vi "dummy_read.vi"(4 "ViStatusOut 2":T2, 5 "InterfaceInfoOut 2":T1, 6 "SyncType3000":enum16{"none", "TTL", "TTL_kadr", "analog"}(ring), 7 "Ctrl Reference":refnum<vi>) -> (0 "ViStatusOut":T2, 2 "InterfaceInfoOut":T1)   [LabVIEW 2010]
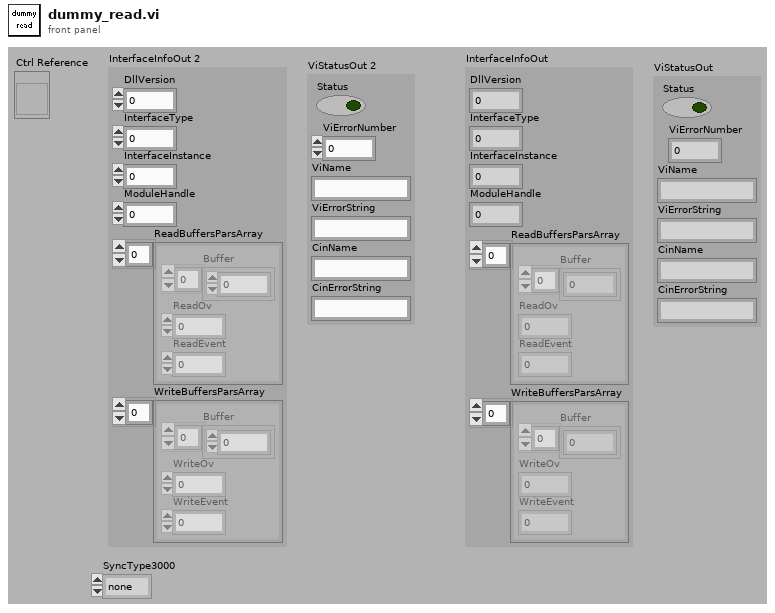
[diagram p1: front panel]
types:
  T1 = cluster{"DllVersion":u32, "InterfaceType":u32, "InterfaceInstance":u32, "ModuleHandle":u32, "ReadBuffersParsArray":cluster{"Buffer":i16[], "ReadOv":u32, "ReadEvent":u32}[], "WriteBuffersParsArray":cluster{"Buffer":i16[], "WriteOv":u32, "WriteEvent":u32}[]}
  T2 = cluster{"Status":bool, "ViErrorNumber":u32, "ViName":string, "ViErrorString":string, "CinName":string, "CinErrorString":string}
  T3 = cluster{"size":u16, "InputEnabled":bool, "CorrectionEnabled":bool, "InputClockSource":u16, "InputType":u16, "SynchroType":u16, "SynchroAdType":u16, "SynchroAdMode":u16, "SynchroAdChannel":u16, "SynchroAdPorog":i16, "ChannelsQuantity":u16, "ControlTable":u16[], "InputFifoBaseAddress":u16, "InputFifoLength":u16, "InputRate":dbl, "InterKadrDelay":dbl, "ChannelRate":dbl, "AdcOffsetCoefArray":dbl[], "AdcScaleCoefArray":dbl[], "BuffersLengthArray":u32[]}
  T4 = cluster{"index":i32, "BufferLength":u32, "RequestStatus":bool}
  T5 = cluster{"ReadBufferIndex":u32, "NumberOfWordsToRead":u32, "RequestStatus":bool}
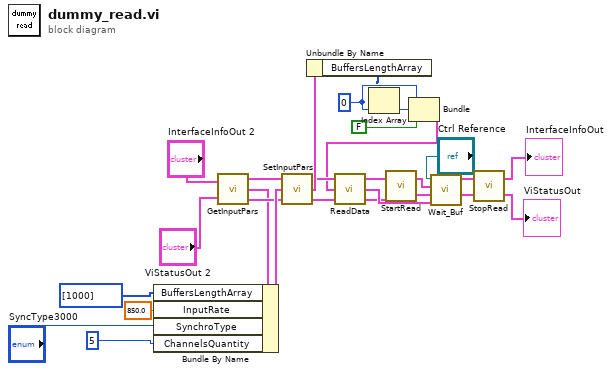
[diagram p0: block diagram]
diagram:
  w26 = 0 ("index")
  n1 = call "GetInputPars.vi"("InterfaceInfoIn"="InterfaceInfoOut 2", "ViStatusIn"="ViStatusOut 2") -> ("InterfaceInfoOut"=w9:T1, "InputParsOut"=w7:T3, "ViStatusOut"=w12:T2)
  n2 = Bundle By Name(cluster=w7, "BuffersLengthArray"=u32[] [1000] ("appended array"), "InputRate"=850.0, "SynchroType"="SyncType3000", "ChannelsQuantity"=u16 5) -> (w15:T3)
  n3 = call "SetInputPars.vi"("ViStatusIn"=w12, "InputParsIn"=w15, "InterfaceInfoIn"=w9) -> ("ViStatusOut"=w3:T2, "InputParsOut"=w24:T3, "InterfaceInfoOut"=w6:T1)
  n4 = Unbundle By Name(w24) -> ("BuffersLengthArray"=w25:u32[])
  n5 = Index Array(array=w25, index=w26) -> (element=w27:u32)
  n6 = Bundle("index"=w26, "BufferLength"=w27, "RequestStatus"=FALSE) -> (w1:T4)  [unwired: 1 in]
  n7 = call "ReadData.vi"("ViStatusIn"=w3, "ReadParsIn"=w1, "InterfaceInfoIn"=w6) -> ("ViStatusOut"=w2:T2, "ReadParsOut"=w4:T5, "InterfaceInfoOut"=w5:T1)
  n8 = call "StartRead.vi"("ViStatusIn"=w2, "InterfaceInfoIn"=w5) -> ("ViStatusOut"=w13:T2, "InterfaceInfoOut"=w10:T1)
  n9 = call "Wait_Buf.vi"("ReadParsIn"=w4, "ViStatusIn"=w13, "InterfaceInfoIn"=w10, "reference"="Ctrl Reference") -> ("ViStatusOut"=w14:T2, "InterfaceInfoOut"=w11:T1)  [unwired: 2 in, 1 out]
  n10 = call "StopRead.vi"("ViStatusIn"=w14, "InterfaceInfoIn"=w11) -> ("ViStatusOut"=→"ViStatusOut":T2, "InterfaceInfoOut"=→"InterfaceInfoOut":T1)
